vi "Read SGL.vi"(8 "error in (no error)":errorcluster, 9 "Type":sgl, 10 "Tag":string, 11 "Var Bus in":refnum<class "Omni_Bus.lvclass">) -> (0 "error out":errorcluster, 2 "Numeric":sgl, 3 "Var Bus out":refnum<class "Omni_Bus.lvclass">)   [LabVIEW 2021, in "Omni_Bus.lvclass"]
uses:
  Omni_Bus.lvclass
  Omni_Bus.lvclass/Omni_Bus.ctl
  <vilib>/TSA/Abstract Data Classes/Abs_Types/Single Float/Abs_Single Float.lvclass
  C:/Program Files (x86)/National Instruments/LabVIEW 2021/vi.lib/TSA/Abstract Data Classes/Abs_Types/Floating Point/Abs_Floating Point.lvclass
  C:/Program Files (x86)/National Instruments/LabVIEW 2021/vi.lib/TSA/Abstract Data Classes/Abs_Types/Numeric/Abs_Numeric.lvclass
  C:/Program Files (x86)/National Instruments/LabVIEW 2021/vi.lib/TSA/Abstract Data Classes/Abs_Types/Value/Abs_Value.lvclass
  C:/Program Files (x86)/National Instruments/LabVIEW 2021/vi.lib/TSA/Abstract Data Classes/Abs_Types/Type/Abs_Type.lvclass
  C:/Program Files (x86)/National Instruments/LabVIEW 2021/vi.lib/TSA/Abstract Data Classes/Abs_Types/Single Float/Abs_Single Float.lvclass
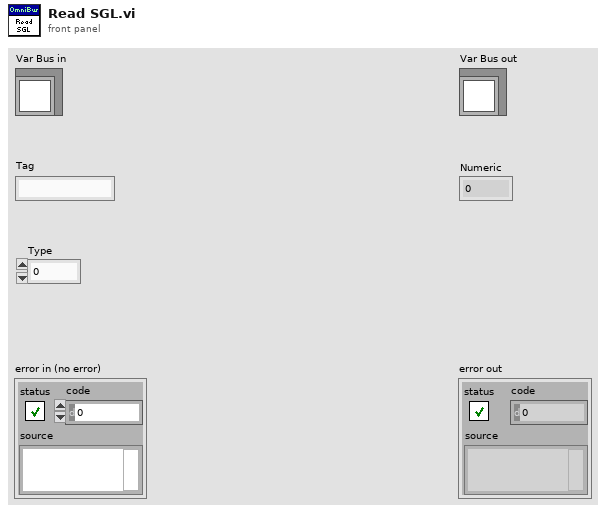
[diagram p1: front panel]
types:
  T1 = typedef "Abs_Single Float.lvclass/Type.ctl" = sgl
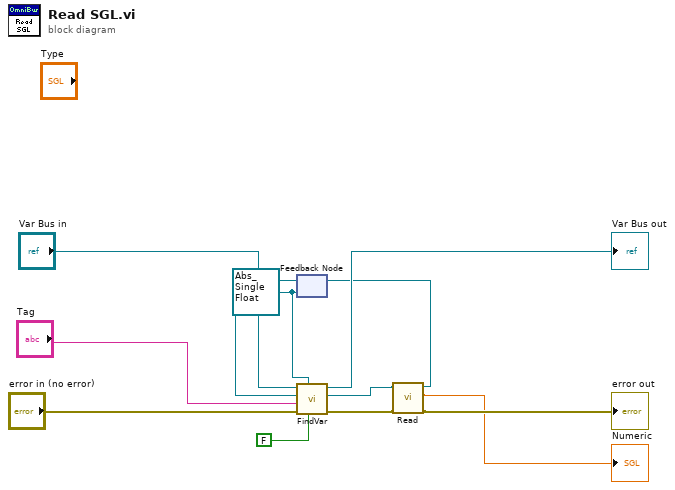
[diagram p0: block diagram]
diagram:
  w1 = refnum<class "Abs_Single Float.lvclass"> refnum ("Double Float.lvclass_340760 out")
  n1 = feedback #1(w1) -> (w6:refnum<class "Abs_Single Float.lvclass">)
  n2 = call "FindVar.vi"("Write?"=FALSE, "Abs_Type"=w1, "error in (no error)"="error in (no error)", "Tag"="Tag", "Abs_Type Default"=w6, "Var Bus in"="Var Bus in") -> ("error out"=w5:errorcluster, "Abs_Type Found"=w4:refnum<class "Abs_Single Float.lvclass">, "Var Bus out"=→"Var Bus out":refnum<class "Omni_Bus.lvclass">)  [unwired: 2 in, 1 out]
  n3 = call-dynamic "Read.vi"("error in (no error)"=w5, "Double Float.lvclass_340760 in"=w4) -> ("error out"=→"error out":errorcluster, "Value"=→"Numeric":T1, "Double Float.lvclass_340760 out"=w3:refnum<class "Abs_Single Float.lvclass">)  [unwired: 7 in]
  n4 = feedback-in #1(w3) -> ()
